vi "Lb_Control.vi"() -> ()   [LabVIEW 2020]
uses:
  <vilib>/Instr/_visa.llb/VISA Configure Serial Port (Instr).vi
panel:
  out "Waveform Chart":dbl(graph)
  in  "VISA resource name":refnum<visa-resource-name>
  in  "On":bool
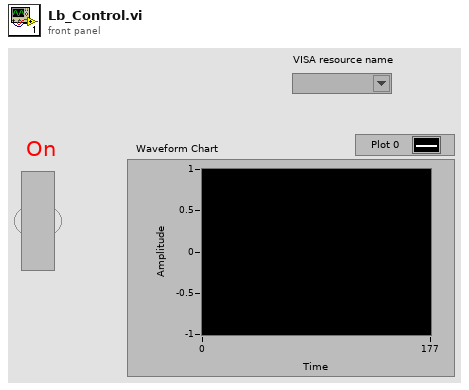
[diagram p1: front panel]
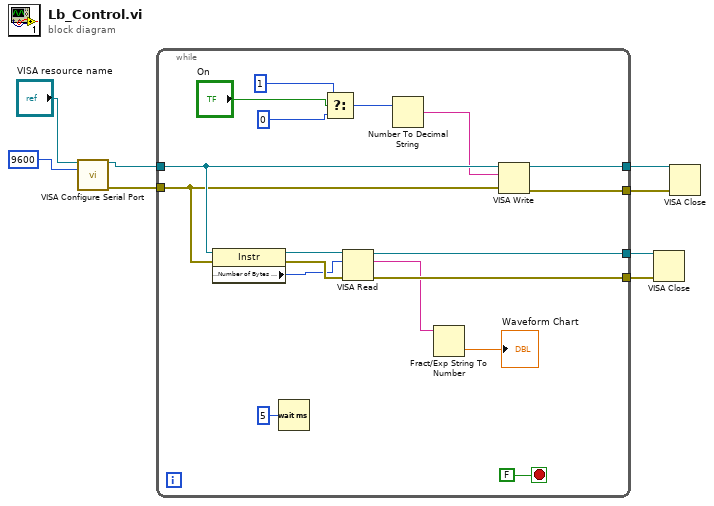
[diagram p0: block diagram]
diagram:
  n1 = call-poly "VISA Configure Serial Port"("VISA resource name"="VISA resource name", "baud rate (9600)"=u32 9600) -> ("VISA resource name out"=w8:refnum<visa-resource-name>, "error out"=w6:errorcluster)  [unwired: 12 in]
  n2 = while {
    tunnel: w8 -> [w18]
    tunnel: [w26] -> w7
    tunnel: w6 -> [w17]
    tunnel: [w25] -> w5
    tunnel: [w22] -> w2
    tunnel: [w20] -> w1
    stop <- FALSE stop-if-true
    n3 = property class="Instr"(reference=w18, error in=w17) -> (reference out=w23:refnum<visa-resource-name>, error out=w21:errorcluster, "Serial Settings:Number of Bytes at Serial Port"=w19:u32)
    n4 = Wait (ms)(milliseconds to wait=u32 5) -> ()  [unwired: 1 out]
    n5 = Select(t=1, s="On", f=0) -> (s? t:f=w11:i32)
    n6 = VISA Read(VISA resource name=w23, byte count=w19, error in (no error)=w21) -> (VISA resource name out=w22:refnum<visa-resource-name>, read buffer=w16:string, error out=w20:errorcluster)  [unwired: 1 out]
    n7 = Number To Decimal String(number=w11) -> (decimal integer string=w10:string)  [unwired: 1 in]
    n8 = Fract/Exp String To Number(string=w16) -> (number=→"Waveform Chart":dbl)  [unwired: 3 in, 1 out]
    n9 = VISA Write(VISA resource name=w18, write buffer=w10, error in (no error)=w17) -> (VISA resource name out=w26:refnum<visa-resource-name>, error out=w25:errorcluster)  [unwired: 1 out]
  }
  n10 = VISA Close(VISA resource name=w2, error in (no error)=w1) -> ()  [unwired: 1 out]
  n11 = VISA Close(VISA resource name=w7, error in (no error)=w5) -> ()  [unwired: 1 out]
